vi "Cochlear Function Test Suite - Copy.vi"() -> ()   [LabVIEW 2020]
uses:
  CFTS SubVIs/CFTS-Globals.vi
  VsEP VIs/VsEP I-O Calibrator.vi
  ABR VIs/ABR Main Panel.vi
  ABR VIs/ABR3 Main Panel.vi
  CAPTH VIs/CAPTH Main Panel.vi
  DPOAE VIs/DP I-O (F1L1).vi
  DPOAE VIs/DP I-O Main Panel.vi
  Digital Exposure VIs/Digital Exposure Controller.vi
  RW Noise VIs/RW Noise VIs/RW Noise Controller.vi
  VsEP VIs/VsEP I-O Controller.vi
  DPOAE VIs/DP Analysis Panel.vi
  epl-vi-lib/Connection VIs/Connection Manager.vi
  System Test VIs/System Test.vi
  epl-cal-vi-lib/Calibrate Probe Tube.vi
  CAP Forward Masking/CAP Forward Masking.vi
  SFOAE VIs/SFOAE Main Panel.vi
  RW Noise VIs/PSTR VIs/PSTR Controller.vi
  epl-vi-lib/Utility VIs/File IO VIs/Configuration File Wrapper VIs/Config-Read Key (Boolean).vi
  epl-cal-vi-lib/Calibrate In Ear.vi
  <vilib>/Utility/miscctls.llb/LVStringsAndValuesArrayTypeDef_U16.ctl
  epl-vi-lib/Utility VIs/File IO VIs/Configuration File Wrapper VIs/Config-Read Key (string).vi
  CFTS SubVIs/CFTS-Experiment State.ctl
panel:
  in  "Other OAE":u16(ring) items=["Other OAE", "SFOAE", "SOAE"]
  in  "Undo":bool
  in  "Apply":bool
  in  "RW":u16(ring) items=["RW", "RW Noise", "PSTR"]
  in  "Other ABR":u16(ring) items=["Other ABR", "Masked ABR", "Fast ABR"]
  in  "Vitals":bool
  in  "Left":u16(ring) items=["---", "ABI-L", "ABI-R", "Insert Left", "Insert Right", "Left", "Right", "SN24", "SN31", "SN32", "SN36", "SN40", "SN41", "SN42"]
  in  "Right":u16(ring) items=["---", "ABI-L", "ABI-R", "Insert Left", "Insert Right", "Left", "Right", "SN24", "SN31", "SN32", "SN36", "SN40", "SN41", "SN42"]
  in  "CAP FM":bool caption="Boolean"
  in  "Options":bool
  in  "Expt State":T1 caption="Setup Options"
  in  "Help":bool
  in  "DP analysis":bool caption="Boolean"
  in  "Exposure":bool caption="Boolean"
  in  "System Test":bool
  in  "VsEP":bool caption="Boolean"
  out "VsEP Run#":i16
  in  "Connections":bool
  in  "VsEP Cal":bool
  in  "CAPTH":bool caption="Boolean"
  out "DP Run#":i16
  out "ABR Run#":i16
  out "CAP Run #":i16
  out "Data Folder":path
  in  "ABR":bool caption="Boolean"
  in  "DP I/O":bool caption="Boolean"
  in  "Calibrate in ear":bool
  in  "Calibrate probe tube":bool
  in  "Quit":bool caption="Boolean"
  # "EPL Cochlear Function Test Suite"
  # "Calibration"
  # "Measurements"
  # "Acoustic Systems"
  # "CTRL-A toggles advanced menu"
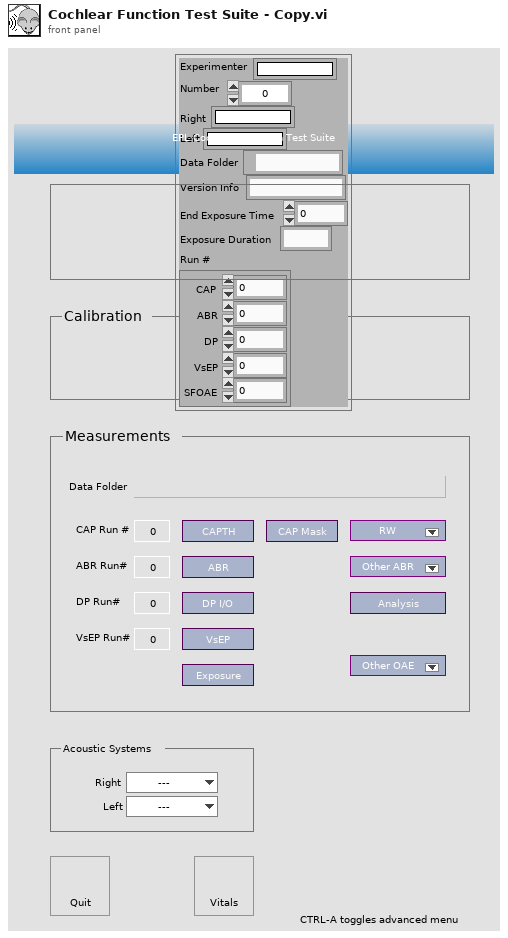
[diagram p1: front panel]
types:
  T1 = typedef "CFTS-Experiment State.ctl" = cluster{"Experimenter":string, "Number":u32, "Right":string, "Left":string, "Data Folder":path, "Version Info":string, "End Exposure Time":dbl, "Exposure Duration":string, "Run #":cluster{"CAP":i32, "ABR":i32, "DP":i32, "VsEP":i32, "SFOAE":i32}}
  T2 = typedef "LVStringsAndValuesArrayTypeDef_U16.ctl" = cluster{"String":string, "Value":u16}[]
  T3 = cluster{"CAP RUN #":refnum<vi>, "ABR RUN #":refnum<vi>, "DP RUN #":refnum<vi>, "VsEP RUN #":refnum<vi>}
  T4 = typedef "CFTS-Experiment State.ctl" = cluster{"Experimenter":string, "Number":u32, "Right":string, "Left":string, "Data Folder":path, "State File":path, "Version Info":string, "End Exposure Time":dbl, "Exposure Duration":string, "Run #":cluster{"CAP":i16, "ABR":i16, "DP":i16, "VsEP":i16, "MeasSeq":i16, "SubSeq":i16, "SFOAE":i16}}
  T5 = typedef "CFTS-Options.ctl" = cluster{"DP Artifact Rejection":bool, "Monitor vital signs ":bool, "Extension":string}
  T6 = cluster{"Experimenter":string, "Number":u32, "Right":string, "Left":string, "Data Folder":path, "State File":path, "Version Info":string, "End Exposure Time":dbl, "Exposure Duration":string, "Run #":cluster{"CAP":i16, "ABR":i16, "DP":i16, "VsEP":i16, "MeasSeq":i16, "SubSeq":i16, "SFOAE":i16}}
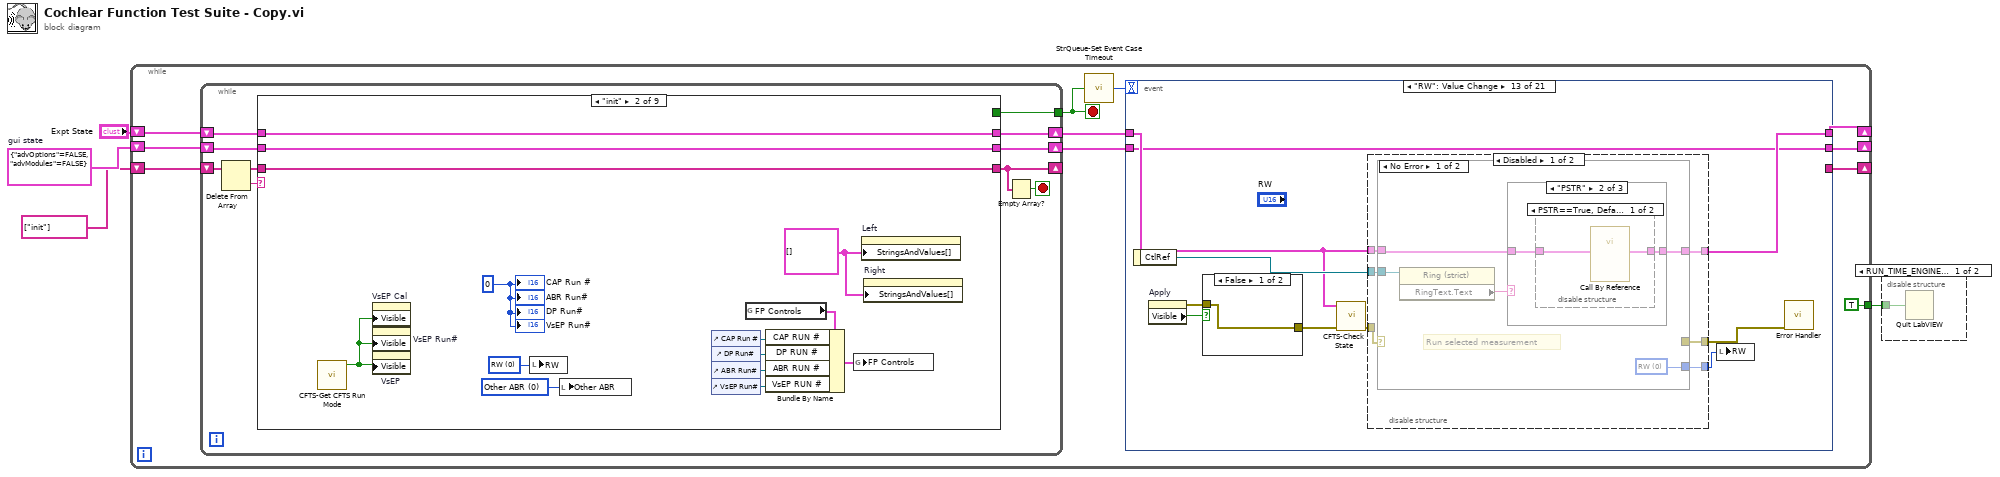
[diagram p0: block diagram]
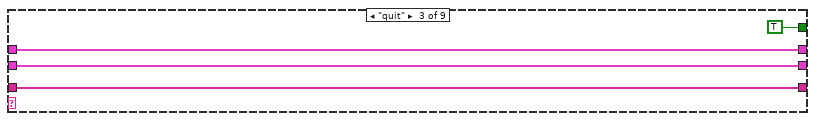
[diagram p3: hidden frame]
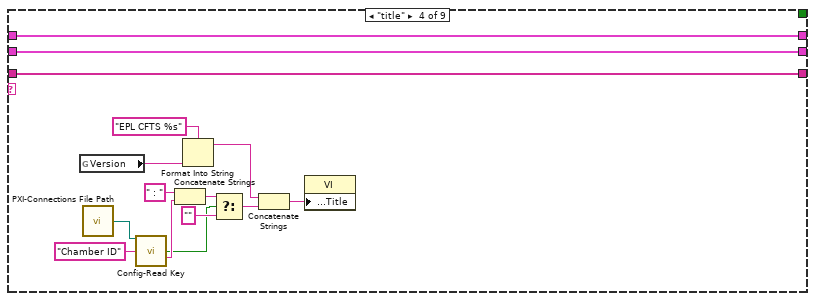
[diagram p4: hidden frame]
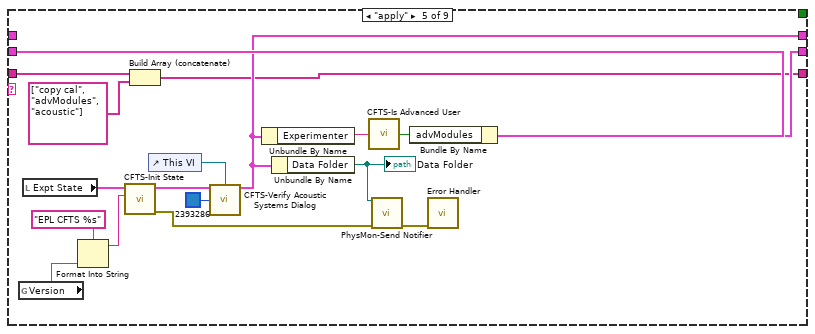
[diagram p5: hidden frame]
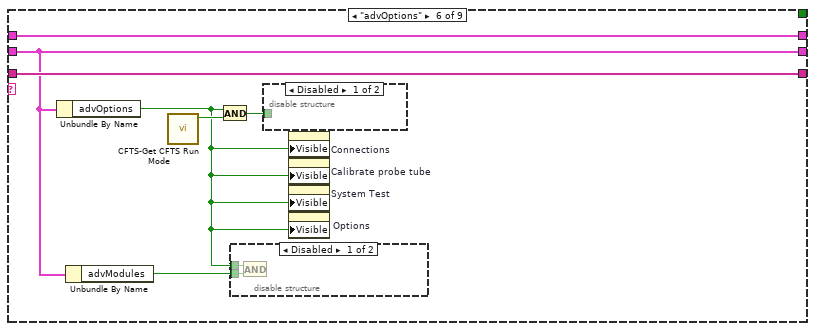
[diagram p6: hidden frame]
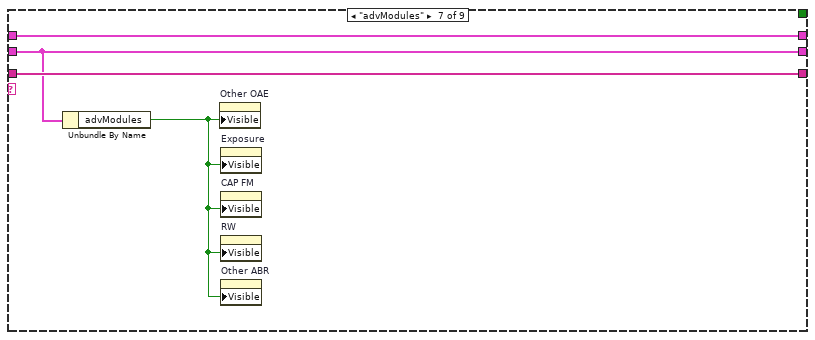
[diagram p9: hidden frame]
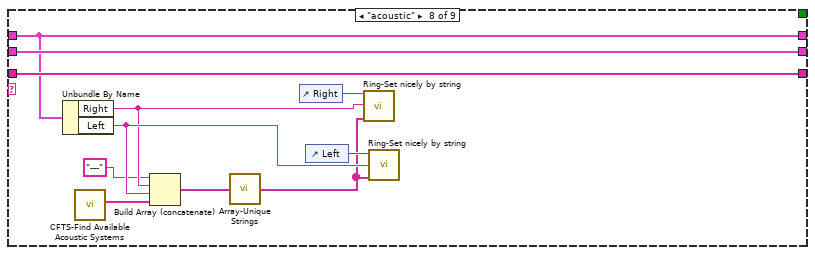
[diagram p10: hidden frame]
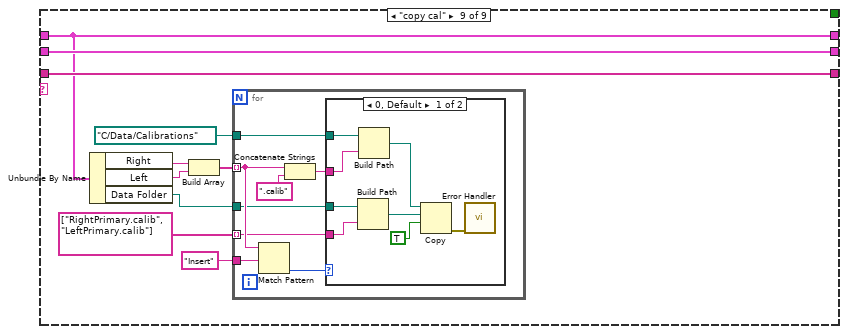
[diagram p11: hidden frame]
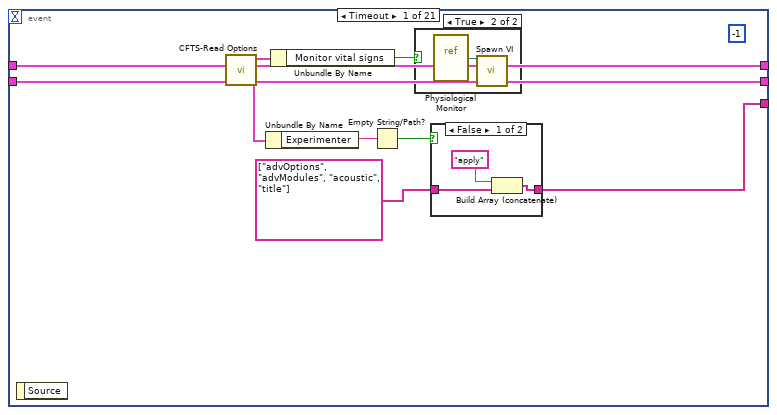
[diagram p13: hidden frame]
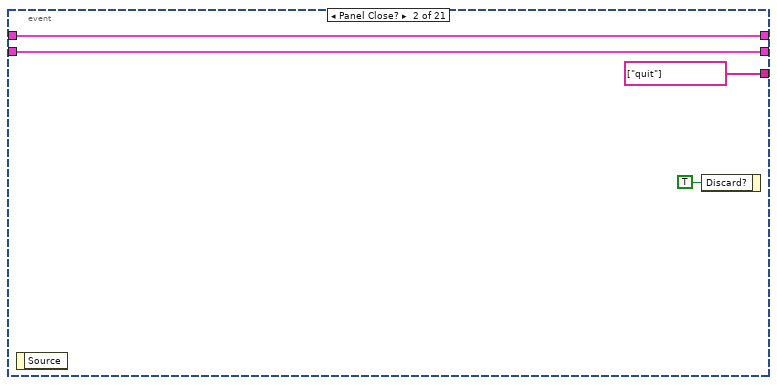
[diagram p16: hidden frame]
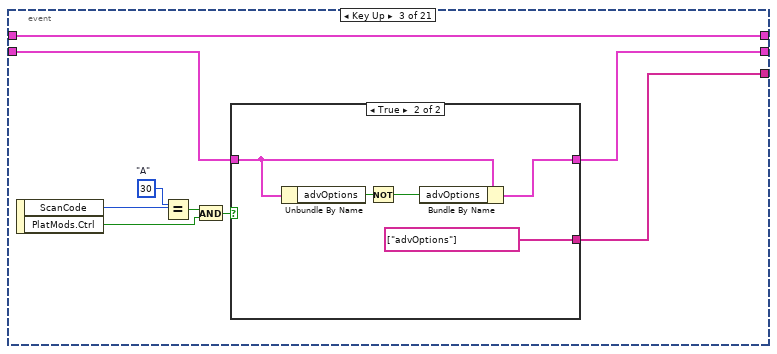
[diagram p17: hidden frame]
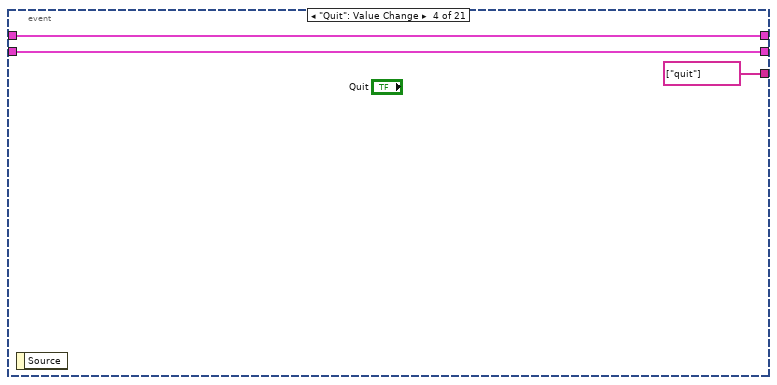
[diagram p19: hidden frame]
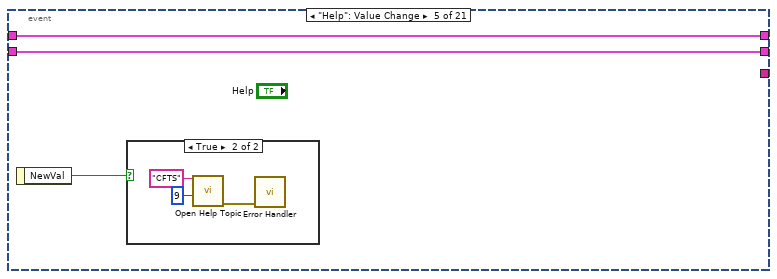
[diagram p20: hidden frame]
diagram:
  w2 = cluster{"advOptions":bool, "advModules":bool} {"advOptions"=FALSE, "advModules"=FALSE}  # gui state
  n1 = while {
    shift-right: [w10] -> _
    shift-left: "Expt State" -> [w14]
    tunnel: [TRUE] -> w3
    shift-right: [w9] -> _
    shift-left: w2 -> [w13]
    shift-right: [w5] -> _
    shift-left: string[] ["init"] ("Array") -> [w8]
    stop <- w6 stop-if-true
    n2 = while {
      shift-right: [w22] -> _
      shift-left: w8 -> [w25]
      tunnel: [w20] -> w6
      shift-right: [w19] -> w12
      shift-left: w14 -> [w18]
      shift-right: [w16] -> w11
      shift-left: w13 -> [w17]
      stop <- w21 stop-if-true
      n3 = Delete From Array(array=w25) -> (deleted portion=w23:string, array with subset deleted=w24:string[])  [unwired: 2 in]
      n4 = case shown="\"init\"" w23 {
        tunnel: w24 -> [w28 w42 w46 w61 w79 w86 w94 w105 w115]
        tunnel: [w28 w42 w46 w61 w67 w86 w94 w105 w115] -> w22
        tunnel: [_ _ TRUE _ _ _ _ _ _] -> w20
        tunnel: [w27 w41 w44 w60 w70 w85 w93 w103 w113] -> w19
        tunnel: w18 -> [w27 w41 w44 w60 _ w85 w93 w103 w113]
        tunnel: w17 -> [w26 w40 w43 w59 w78 w82 w92 w104 w114]
        tunnel: [w26 w40 w43 w59 w69 w82 w92 w104 w114] -> w16
        frame "", Default {
        }
        frame "init" {
          w29 = T2 [] ("Strings And Values []")
          w36 = i16 0 ("CAP RUN #")
          w38 = u16 0 items=["RW", "RW Noise", "PSTR"] ("RW")
          w37 = u16 0 items=["Other ABR", "Mask ABR", "Fast ABR"] ("Other ABR")
          n5 = call "CFTS-Get CFTS Run Mode.vi"() -> ("EPL Internal?"=w39:bool)  [unwired: 10 in, 1 out]
          n6 = property on="VsEP Cal" class="Bool"("Visible"=w39) -> ()  [unwired: 2 in, 2 out]
          n7 = property on="VsEP Run#" class="DigNum (strict)"("Visible"=w39) -> ()  [unwired: 2 in, 2 out]
          n8 = property on="VsEP" class="Bool"("Visible"=w39) -> ()  [unwired: 2 in, 2 out]
          n9 = local write "RW"(w38) -> ()
          n10 = local write "Other ABR"(w37) -> ()
          n11 = control-ref of="CAP Run #"() -> (w35:refnum<vi>)
          n12 = control-ref of="DP Run#"() -> (w34:refnum<vi>)
          n13 = control-ref of="ABR Run#"() -> (w33:refnum<vi>)
          n14 = control-ref of="VsEP Run#"() -> (w32:refnum<vi>)
          n15 = global read "CFTS-Globals.vi" "FP Controls"() -> (w30:T3)
          n16 = Bundle By Name(cluster=w30, "CAP RUN #"=w35, "DP RUN #"=w34, "ABR RUN #"=w33, "VsEP RUN #"=w32) -> (w31:T3)
          n17 = global write "CFTS-Globals.vi" "FP Controls"(w31) -> ()
          n18 = property on="Left" class="Ring (strict)"("StringsAndValues[]"=w29) -> ()  [unwired: 2 in, 2 out]
          n19 = property on="Right" class="Ring (strict)"("StringsAndValues[]"=w29) -> ()  [unwired: 2 in, 2 out]
          "CAP Run #" <- w36
          "ABR Run#" <- w36
          "DP Run#" <- w36
          "VsEP Run#" <- w36
        }
        frame "quit" {
        }
        frame "title" {
          n20 = global read "CFTS-Globals.vi" "Version"() -> (w47:string)
          n21 = call "PXI-Connections File Path.vi"() -> ("Path"=w58:path)  [unwired: 1 in]
          n22 = call-poly "Config-Read Key.vi"("configuration file path"=w58, "key"="Chamber ID" ("string")) -> ("found?"=w50:bool, "value"=w57:string)  [unwired: 10 in, 2 out]
          n23 = Concatenate Strings(" : " ("string"), w57) -> (w49:string)
          n24 = Format Into String(format string="EPL CFTS %s" ("string"), w47) -> (resulting string=w51:string)  [unwired: 2 in, 1 out]
          n25 = Select(t=w49, s=w50, f="") -> (s? t:f=w55:string)
          n26 = Concatenate Strings(w51, w55) -> (w52:string)
          n27 = property class="VI"("Front Panel.Title"=w52) -> ()  [unwired: 2 in, 2 out]
        }
        frame "apply" {
          n28 = global read "CFTS-Globals.vi" "Version"() -> (w62:string)
          n29 = local read "Expt State"() -> (w73:T1)
          n30 = Format Into String(format string="EPL CFTS %s" ("string"), w62) -> (resulting string=w63:string)  [unwired: 2 in, 1 out]
          n31 = call "CFTS-Init State.vi"("CFTS Version"=w63, "Experiment State (in)"=w73) -> ("error out"=w71:errorcluster, "Experiment State (out)"=w75:T4)  [unwired: 8 in]
          n32 = Build Array (concatenate)(w79, string[] ["copy cal", "advModules", "acoustic"]) -> (w67:string[])
          n33 = control-ref of="This VI"() -> (w76:refnum<vi>)
          n34 = call "CFTS-Verify Acoustic Systems Dialog.vi"("Expt State"=w75, "center on"=w76, "color"=u32 2393286) -> ("Cluster out"=w70:T1)  [unwired: 11 in, 1 out]
          n35 = Unbundle By Name(w70) -> ("Experimenter"=w74:string)
          n36 = Unbundle By Name(w70) -> ("Data Folder"=w65:path)
          "Data Folder" <- w65
          n37 = call "CFTS-Is Advanced User.vi"("Experimenter"=w74) -> ("Advanced user"=w68:bool)
          n38 = call "PhysMon-Send Notifier.vi"("Path"=w65, "error in (no error)"=w71) -> ("error out"=w72:errorcluster)  [unwired: 13 in]
          n39 = Bundle By Name(cluster=w78, "advModules"=w68) -> (w69:cluster{"advOptions":bool, "advModules":bool})
          n40 = call "Error Handler.vi"("error in (no error)"=w72) -> ()  [unwired: 13 in, 2 out]
        }
        frame "advOptions" {
          n41 = Unbundle By Name(w82) -> ("advOptions"=w81:bool)
          n42 = Unbundle By Name(w82) -> ("advModules"=w80:bool)
          n43 = call "CFTS-Get CFTS Run Mode.vi"() -> ("EPL Internal?"=w83:bool)  [unwired: 10 in, 1 out]
          n44 = And(x=w81, y=w83) -> (x .and. y?=w84:bool)
          n45 = disable-structure shown="Disabled" {
            disable-tunnel: w81 -> [w89 _]
            disable-tunnel: w80 -> [w88 _]
            frame Disabled {
              n46 = And(x=w89, y=w88) -> (x .and. y?=w90:bool)
            }
            frame Enabled {
            }
          }
          n47 = disable-structure shown="Disabled" {
            disable-tunnel: w84 -> [w87 _]
            frame Disabled {
            }
            frame Enabled {
            }
          }
          n48 = property on="Connections" class="Bool"("Visible"=w81) -> ()  [unwired: 2 in, 2 out]
          n49 = property on="Calibrate probe tube" class="Bool"("Visible"=w81) -> ()  [unwired: 2 in, 2 out]
          n50 = property on="System Test" class="Bool"("Visible"=w81) -> ()  [unwired: 2 in, 2 out]
          n51 = property on="Options" class="Bool"("Visible"=w81) -> ()  [unwired: 2 in, 2 out]
        }
        frame "advModules" {
          n52 = Unbundle By Name(w92) -> ("advModules"=w91:bool)
          n53 = property on="Other OAE" class="Ring (strict)"("Visible"=w91) -> ()  [unwired: 2 in, 2 out]
          n54 = property on="Exposure" class="Bool"("Visible"=w91) -> ()  [unwired: 2 in, 2 out]
          n55 = property on="CAP FM" class="Bool"("Visible"=w91) -> ()  [unwired: 2 in, 2 out]
          n56 = property on="RW" class="Ring (strict)"("Visible"=w91) -> ()  [unwired: 2 in, 2 out]
          n57 = property on="Other ABR" class="Ring (strict)"("Visible"=w91) -> ()  [unwired: 2 in, 2 out]
        }
        frame "acoustic" {
          n58 = Unbundle By Name(w103) -> ("Right"=w98:string, "Left"=w99:string)
          n59 = call "CFTS-Find Available Acoustic Systems.vi"() -> ("Acoustic Systems"=w100:string[])  [unwired: 11 in]
          n60 = Build Array (concatenate)("---", w98, w99, w100) -> (w96:string[])
          n61 = call "Array-Unique Strings.vi"("Strings"=w96) -> ("Unique strings"=w95:string[])  [unwired: 4 in]
          n62 = control-ref of="Right"() -> (w102:refnum<vi>)
          n63 = control-ref of="Left"() -> (w101:refnum<vi>)
          n64 = call "Ring-Set nicely by string.vi"("Ring in"=w102, "Device"=w98, "Strings []"=w95) -> ()  [unwired: 8 in, 5 out]
          n65 = call "Ring-Set nicely by string.vi"("Ring in"=w101, "Device"=w99, "Strings []"=w95) -> ()  [unwired: 8 in, 5 out]
        }
        frame "copy cal" {
          n66 = Unbundle By Name(w113) -> ("Right"=w112:string, "Left"=w111:string, "Data Folder"=w107:path)
          n67 = Build Array(w112, w111) -> (w110:string[])
          n68 = for {
            tunnel: w110 -> [w121] mode=indexing
            tunnel: "Insert" ("regular expression") -> [w123]
            tunnel: path "C:/Data/Calibrations" ("path") -> [w118]
            tunnel: w107 -> [w117]
            tunnel: string[] ["RightPrimary.calib", "LeftPrimary.calib"] ("regular expression") -> [w116] mode=indexing
            n69 = Match Pattern(string=w121, regular expression=w123) -> (offset past match=w122:i32)  [unwired: 1 in, 3 out]
            n70 = Concatenate Strings(w121, ".calib") -> (w119:string)
            n71 = case shown="0, Default" w122 {
              tunnel: w119 -> [w128 _]
              tunnel: w118 -> [w129 _]
              tunnel: w117 -> [w126 _]
              tunnel: w116 -> [w125 _]
              frame 0, Default {
                n72 = Build Path(base path=w126, name or relative path=w125) -> (appended path=w131:path)
                n73 = Build Path(base path=w129, name or relative path=w128) -> (appended path=w127:path)
                n74 = Copy(9:TRUE ("overwrite (F)"), 10:w131, 11:w127) -> (0:w130:errorcluster)  [unwired: 2 in, 2 out]
                n75 = call "Error Handler.vi"("error in (no error)"=w130) -> ()  [unwired: 13 in, 2 out]
              }
              frame -1 {
              }
            }
          }
        }
      }
      n76 = Empty Array?(array=w22) -> (empty?=w21:bool)
    }
    n77 = call "StrQueue-Set Event Case Timeout.vi"("Quit"=w6) -> ("timeout"=w7:i32)  [unwired: 14 in]
    n78 = event shown="[12] \"RW\": Value Change" {
      selector: _ -> [_ _ _ _ _ _ _ _ _ _ _ _ _ _ _ _ _ _ _ _ _]
      dyn-events: _ -> [_ _ _ _ _ _ _ _ _ _ _ _ _ _ _ _ _ _ _ _ _]
      timeout: w7 -> [_ _ _ _ _ _ _ _ _ _ _ _ _ _ _ _ _ _ _ _ _]
      tunnel: w12 -> [w136 w147 w152 w166 w169 w175 w178 w184 w189 w191 w201 w210 w260 w294 w325 w355 w359 w365 w372 w377 w383]
      tunnel: [w136 w147 w152 w166 w169 w175 w178 w184 w188 w191 w201 w216 w266 w300 w331 w355 w359 w362 w372 w377 w383] -> w10
      tunnel: [w132 string[] ["quit"] w149 string[] ["quit"] _ _ string[] ["apply"] _ _ _ _ _ _ _ _ _ _ string[] ["acoustic", "title"] _ string[] ["acoustic"] _] -> w5
      tunnel: [w137 w145 w150 w164 w167 w173 w177 w181 w185 w190 w200 w209 w258 w292 w323 w354 w358 w361 w371 w376 w382] -> w9
      tunnel: w11 -> [w137 w145 w151 w164 w167 w173 w177 w181 w185 w190 w200 w209 w258 w292 w323 w354 w358 w361 w371 w376 w382]
      event Timeout {
        (unwired) -1
        n79 = event-data() -> ()  [unwired: 1 in, 1 out]
        n80 = call "CFTS-Read Options.vi"() -> ("CFTS Options"=w139:T5)  [unwired: 10 in, 1 out]
        n81 = Unbundle By Name(w136) -> ("Experimenter"=w135:string)
        n82 = Unbundle By Name(w139) -> ("Monitor vital signs"=w138:bool)
        n83 = Empty String/Path?(string/path=w135) -> (empty?=w134:bool)
        n84 = case shown="True" w138 {
          frame False {
          }
          frame True {
            n85 = vi-ref "Physiological Monitor.vi"() -> (w144:refnum<vi>)
            n86 = call "Spawn VI.vi"("VI reference"=w144) -> ()  [unwired: 9 in, 2 out]
          }
        }
        n87 = case shown="False" w134 {
          tunnel: string[] ["advOptions", "advModules", "acoustic", "title"] -> [w142 w143]
          tunnel: [w141 w143] -> w132
          frame False {
            n88 = Build Array (concatenate)("apply", w142) -> (w141:string[])
          }
          frame True {
          }
        }
      }
      event Panel Close? {
        n89 = event-data() -> ()  [unwired: 1 in, 1 out]
        n90 = event-data("Discard?"=TRUE) -> ()  [unwired: 1 in, 1 out]
      }
      event Key Up {
        w156 = i16 30  # "A"
        n91 = event-data() -> ("ScanCode"=w157:i16, "PlatMods.Ctrl"=w154:bool)  [unwired: 1 in]
        n92 = Equal?(x=w156, y=w157) -> (x = y?=w155:bool)
        n93 = And(x=w155, y=w154) -> (x .and. y?=w153:bool)
        n94 = case shown="True" w153 {
          tunnel: w151 -> [w158 w163]
          tunnel: [w158 w160] -> w150
          tunnel: [_ string[] ["advOptions"]] -> w149
          frame False {
          }
          frame True {
            n95 = Unbundle By Name(w163) -> ("advOptions"=w162:bool)
            n96 = Not(x=w162) -> (.not. x?=w161:bool)
            n97 = Bundle By Name(cluster=w163, "advOptions"=w161) -> (w160:cluster{"advOptions":bool, "advModules":bool})
          }
        }
      }
      event "Quit": Value Change {
        n98 = event-data() -> ()  [unwired: 1 in, 1 out]
      }
      event "Help": Value Change {
        n99 = event-data() -> ("NewVal"=w168:bool)  [unwired: 1 in]
        n100 = case shown="True" w168 {
          frame False {
          }
          frame True {
            n101 = call "Open Help Topic.vi"("Help file"="CFTS", "HelpId"=9) -> ("error out"=w171:errorcluster)  [unwired: 13 in]
            n102 = call "Error Handler.vi"("error in (no error)"=w171) -> ()  [unwired: 13 in, 2 out]
          }
        }
      }
      event Value Change {
        w174 = TRUE ("Visible")
        n103 = event-data() -> ()  [unwired: 1 in, 1 out]
        n104 = property on="Undo" class="Bool"("Visible"=w174) -> ()  [unwired: 2 in, 2 out]
        n105 = property on="Apply" class="Bool"("Visible"=w174) -> ()  [unwired: 2 in, 2 out]
      }
      event "Apply": Value Change {
        w179 = FALSE
        n106 = event-data() -> ()  [unwired: 1 in, 1 out]
        n107 = property on="Apply" class="Bool"("Visible"=w179) -> (error out=w180:errorcluster)  [unwired: 2 in, 1 out]
        n108 = property on="Undo" class="Bool"(error in=w180, "Visible"=w179) -> ()  [unwired: 1 in, 2 out]
      }
      event "Undo": Value Change {
        w183 = FALSE
        n109 = event-data() -> ()  [unwired: 1 in, 1 out]
        n110 = local write "Expt State"(w184) -> ()
        n111 = property on="Apply" class="Bool"("Visible"=w183) -> (error out=w182:errorcluster)  [unwired: 2 in, 1 out]
        n112 = property on="Undo" class="Bool"(error in=w182, "Visible"=w183) -> ()  [unwired: 1 in, 2 out]
      }
      event "Right", "Left": Value Change {
        n113 = event-data() -> ()  [unwired: 1 in, 1 out]
        n114 = property on="Left" class="Ring (strict)"() -> ("RingText.Text"=w187:string)  [unwired: 2 in, 2 out]
        n115 = property on="Right" class="Ring (strict)"() -> ("RingText.Text"=w186:string)  [unwired: 2 in, 2 out]
        n116 = Bundle By Name(cluster=w189, "Right"=w186, "Left"=w187) -> (w188:T1)
        n117 = call "CFTS-Store Acoustic System IDs.vi"("Left"=w187, "Right"=w186) -> ()  [unwired: 9 in, 1 out]
      }
      event "Calibrate in ear": Value Change {
        n118 = event-data() -> ()  [unwired: 1 in, 1 out]
        n119 = disable-structure shown="Disabled" {
          disable-tunnel: w191 -> [w193 _]
          frame Disabled {
            n120 = call "CFTS-Check State.vi"("Expt State"=w193) -> ("error out"=w194:errorcluster)  [unwired: 10 in]
            n121 = case shown="No Error" w194 {
              selector: w194 -> [_ w199]
              tunnel: w193 -> [w198 _]
              tunnel: [w197 w199] -> w192
              frame No Error {
                n122 = call "PXI-Connections File Path.vi"() -> ("Path"=w196:path)  [unwired: 1 in]
                n123 = call-poly "Config-Read Key.vi"("configuration file path"=w196, "key"="FPL") -> ()  [unwired: 10 in, 4 out]
                n124 = call-by-ref "?"("State"=w198) -> ("error out"=w197:errorcluster)  [unwired: 12 in, 2 out]
              }
              frame Error {
              }
            }
            n125 = call "Error Handler.vi"("error in (no error)"=w192) -> ()  [unwired: 13 in, 2 out]
          }
          frame Enabled {
          }
        }
      }
      event "VsEP Cal": Value Change {
        n126 = event-data() -> ()  [unwired: 1 in, 1 out]
        n127 = disable-structure shown="Disabled" {
          disable-tunnel: w201 -> [w204 _]
          frame Disabled {
            n128 = call "CFTS-Check State.vi"("Expt State"=w204) -> ("error out"=w203:errorcluster)  [unwired: 10 in]
            n129 = Unbundle By Name(w204) -> ("Data Folder"=w205:path)
            n130 = case shown="No Error" w203 {
              selector: w203 -> [w206 w208]
              tunnel: w205 -> [w207 _]
              tunnel: [w206 w208] -> w202
              frame No Error {
                n131 = call-by-ref "?"("Data Folder"=w207) -> ()  [unwired: 13 in, 2 out]
              }
              frame Error {
              }
            }
            n132 = call "Error Handler.vi"("error in (no error)"=w202) -> ()  [unwired: 13 in, 2 out]
          }
          frame Enabled {
          }
        }
      }
      event "DP I/O", "ABR", "CAPTH", "VsEP", "Exposure", "CAP FM": Value Change {
        n133 = event-data() -> ("CtlRef"=w217:refnum<vi>)  [unwired: 1 in]
        n134 = property on="Apply" class="Bool"() -> (error out=w213:errorcluster, "Visible"=w214:bool)  [unwired: 2 in, 1 out]
        n135 = case shown="True" w214 {
          tunnel: w213 -> [w255 _]
          tunnel: [w255 w256] -> w212
          frame False {
          }
          frame True {
            n136 = call <vilib>:"Error Cluster From Error Code.vi"("error code (0)"=5001) -> ("error out"=w256:errorcluster)  [unwired: 8 in]
          }
        }
        n137 = call "CFTS-Check State.vi"("error in (no error)"=w212, "Expt State"=w210) -> ("error out"=w211:errorcluster)  [unwired: 9 in]
        n138 = disable-structure shown="Disabled" {
          disable-tunnel: w217 -> [w222 _]
          disable-tunnel: [w221 _] -> w216
          disable-tunnel: [w220 _] -> w215
          disable-tunnel: w211 -> [w219 _]
          disable-tunnel: w210 -> [w218 _]
          frame Disabled {
            n139 = case shown="No Error" w219 {
              selector: w219 -> [_ w253]
              tunnel: w222 -> [w226 _]
              tunnel: w218 -> [w224 w254]
              tunnel: [w223 w254] -> w221
              tunnel: [_ w253] -> w220
              frame No Error {
                # "Run selected measurement"
                n140 = property class="Bool"(reference=w226) -> ("Label.Text"=w225:string)  [unwired: 1 in, 2 out]
                n141 = case shown="\"CAPTH\"" w225 {
                  tunnel: w224 -> [w228 w230 w232 w240 w246 w248 w250 w252]
                  tunnel: [w227 w229 w231 w239 w245 w247 w249 w251] -> w223
                  frame "ABR" {
                    n142 = call-by-ref "?"("State (in)"=w228) -> ("State"=w227:T4)  [unwired: 12 in, 2 out]
                  }
                  frame "CAP FM" {
                    n143 = call-by-ref "?"("State"=w230) -> ("State Out"=w229:T4)  [unwired: 12 in, 2 out]
                  }
                  frame "CAPTH" {
                    n144 = disable-structure shown="Enabled" {
                      disable-tunnel: w232 -> [w234 w235]
                      disable-tunnel: [w233 w235] -> w231
                      frame Enabled {
                        n145 = call-by-ref "?"("Expt State (in)"=w234) -> ("State"=w233:T4)  [unwired: 12 in, 2 out]
                      }
                      frame Disabled {
                      }
                    }
                  }
                  frame "DP I/O", Default {
                    n146 = call "PXI-Connections File Path.vi"() -> ("Path"=w236:path)  [unwired: 1 in]
                    n147 = call-poly "Config-Read Key.vi"("configuration file path"=w236, "key"="Advanced DP I-O") -> ("value"=w237:bool)  [unwired: 10 in, 3 out]
                    n148 = case shown="False" w237 {
                      tunnel: w240 -> [w242 w244]
                      tunnel: [w241 w243] -> w239
                      frame True {
                        n149 = call-by-ref "?"("Expt State (in)"=w242) -> ("State"=w241:T4)  [unwired: 12 in, 2 out]
                      }
                      frame False {
                        n150 = call-by-ref "?"("Expt State (in)"=w244) -> ("State"=w243:T4)  [unwired: 12 in, 2 out]
                      }
                    }
                  }
                  frame "Exposure" {
                    n151 = call-by-ref "?"("State in"=w246) -> ("State"=w245:T4)  [unwired: 12 in, 2 out]
                  }
                  frame "Masked ABR" {
                    n152 = call-by-ref "?"("State (in)"=w248) -> ("State"=w247:T4)  [unwired: 12 in, 2 out]
                  }
                  frame "RW Noise" {
                    n153 = call-by-ref "?"("Expt State (in)"=w250) -> ("Expt State"=w249:T4)  [unwired: 12 in, 2 out]
                  }
                  frame "VsEP" {
                    n154 = call-by-ref "?"("Expt State (in)"=w252) -> ("state out"=w251:T4)  [unwired: 12 in, 2 out]
                  }
                }
              }
              frame Error {
              }
            }
          }
          frame Enabled {
          }
        }
        n155 = call "Error Handler.vi"("error in (no error)"=w215) -> ()  [unwired: 13 in, 2 out]
      }
      event "RW": Value Change {
        n156 = event-data() -> ("CtlRef"=w267:refnum<vi>)  [unwired: 1 in]
        n157 = property on="Apply" class="Bool"() -> (error out=w263:errorcluster, "Visible"=w264:bool)  [unwired: 2 in, 1 out]
        n158 = case shown="False" w264 {
          tunnel: w263 -> [w289 _]
          tunnel: [w289 w290] -> w262
          frame False {
          }
          frame True {
            n159 = call <vilib>:"Error Cluster From Error Code.vi"("error code (0)"=5001) -> ("error out"=w290:errorcluster)  [unwired: 8 in]
          }
        }
        n160 = call "CFTS-Check State.vi"("error in (no error)"=w262, "Expt State"=w260) -> ("error out"=w261:errorcluster)  [unwired: 9 in]
        n161 = disable-structure shown="Disabled" {
          disable-tunnel: w267 -> [w273 _]
          disable-tunnel: [w272 _] -> w266
          disable-tunnel: [w271 _] -> w265
          disable-tunnel: w261 -> [w270 _]
          disable-tunnel: w260 -> [w269 _]
          disable-tunnel: [w268 _] -> w259
          frame Disabled {
            n162 = case shown="No Error" w270 {
              selector: w270 -> [_ w287]
              tunnel: w273 -> [w278 _]
              tunnel: w269 -> [w276 w288]
              tunnel: [w275 w288] -> w272
              tunnel: [_ w287] -> w271
              tunnel: [w274 _] -> w268
              frame No Error {
                w274 = u16 0 items=["RW", "RW Noise", "PSTR"] ("RW")
                # "Run selected measurement"
                n163 = property class="Ring (strict)"(reference=w278) -> ("RingText.Text"=w277:string)  [unwired: 1 in, 2 out]
                n164 = case shown="\"PSTR\"" w277 {
                  tunnel: w276 -> [w279 w280 w286]
                  tunnel: [w279 w281 w285] -> w275
                  frame "", Default {
                  }
                  frame "PSTR" {
                    n165 = disable-structure shown="PSTR==True, Default" {
                      disable-tunnel: [w283 w284] -> w281
                      disable-tunnel: w280 -> [w282 w284]
                      frame condition #0 (active) {
                        n166 = call-by-ref "?"("Expt State (in)"=w282) -> ("Expt State"=w283:T4)  [unwired: 12 in, 2 out]
                      }
                      frame condition #1 {
                      }
                    }
                  }
                  frame "RW Noise" {
                    n167 = call-by-ref "?"("Expt State (in)"=w286) -> ("Expt State"=w285:T4)  [unwired: 12 in, 2 out]
                  }
                }
              }
              frame Error {
              }
            }
          }
          frame Enabled {
          }
        }
        n168 = local write "RW"(w259) -> ()
        n169 = call "Error Handler.vi"("error in (no error)"=w265) -> ()  [unwired: 13 in, 2 out]
      }
      event "Other ABR": Value Change {
        n170 = event-data() -> ("CtlRef"=w301:refnum<vi>)  [unwired: 1 in]
        n171 = property on="Apply" class="Bool"() -> (error out=w297:errorcluster, "Visible"=w298:bool)  [unwired: 2 in, 1 out]
        n172 = case shown="True" w298 {
          tunnel: w297 -> [w320 _]
          tunnel: [w320 w321] -> w296
          frame False {
          }
          frame True {
            n173 = call <vilib>:"Error Cluster From Error Code.vi"("error code (0)"=5001) -> ("error out"=w321:errorcluster)  [unwired: 8 in]
          }
        }
        n174 = call "CFTS-Check State.vi"("error in (no error)"=w296, "Expt State"=w294) -> ("error out"=w295:errorcluster)  [unwired: 9 in]
        n175 = disable-structure shown="Disabled" {
          disable-tunnel: w301 -> [w307 _]
          disable-tunnel: [w306 _] -> w300
          disable-tunnel: [w305 _] -> w299
          disable-tunnel: w295 -> [w304 _]
          disable-tunnel: w294 -> [w303 _]
          disable-tunnel: [w302 _] -> w293
          frame Disabled {
            n176 = case shown="No Error" w304 {
              selector: w304 -> [_ w318]
              tunnel: w307 -> [w312 _]
              tunnel: w303 -> [w310 w319]
              tunnel: [w309 w319] -> w306
              tunnel: [_ w318] -> w305
              tunnel: [0 _] -> w302
              frame No Error {
                # "Run selected measurement"
                n177 = property class="Ring (strict)"(reference=w312) -> ("RingText.Text"=w311:string)  [unwired: 1 in, 2 out]
                n178 = case shown="\"Masked ABR\"" w311 {
                  tunnel: w310 -> [w314 w315 w316]
                  tunnel: [w313 w315 w317] -> w309
                  frame "Masked ABR" {
                    n179 = call-by-ref "?"("State (in)"=w314) -> ("State"=w313:T4)  [unwired: 12 in, 2 out]
                  }
                  frame "", Default {
                  }
                  frame "Fast ABR" {
                    n180 = call "Fast ABR.vi"("Expt State (in)"=w316) -> ("Expt State"=w317:T4)  [unwired: 10 in]
                  }
                }
              }
              frame Error {
              }
            }
          }
          frame Enabled {
          }
        }
        n181 = local write "Other ABR"(w293) -> ()
        n182 = call "Error Handler.vi"("error in (no error)"=w299) -> ()  [unwired: 13 in, 2 out]
      }
      event "Other OAE": Value Change {
        n183 = event-data() -> ("CtlRef"=w332:refnum<vi>)  [unwired: 1 in]
        n184 = property on="Apply" class="Bool"() -> (error out=w328:errorcluster, "Visible"=w329:bool)  [unwired: 2 in, 1 out]
        n185 = case shown="True" w329 {
          tunnel: w328 -> [w351 _]
          tunnel: [w351 w352] -> w327
          frame False {
          }
          frame True {
            n186 = call <vilib>:"Error Cluster From Error Code.vi"("error code (0)"=5001) -> ("error out"=w352:errorcluster)  [unwired: 8 in]
          }
        }
        n187 = call "CFTS-Check State.vi"("error in (no error)"=w327, "Expt State"=w325) -> ("error out"=w326:errorcluster)  [unwired: 9 in]
        n188 = disable-structure shown="Disabled" {
          disable-tunnel: w332 -> [w338 _]
          disable-tunnel: [w337 _] -> w331
          disable-tunnel: [w336 _] -> w330
          disable-tunnel: w326 -> [w335 _]
          disable-tunnel: w325 -> [w334 _]
          disable-tunnel: [w333 _] -> w324
          frame Disabled {
            n189 = case shown="No Error" w335 {
              selector: w335 -> [_ w349]
              tunnel: w338 -> [w343 _]
              tunnel: w334 -> [w341 w350]
              tunnel: [w340 w350] -> w337
              tunnel: [_ w349] -> w336
              tunnel: [0 _] -> w333
              frame No Error {
                # "Run selected measurement"
                n190 = property class="Ring (strict)"(reference=w343) -> ("RingText.Text"=w342:string)  [unwired: 1 in, 2 out]
                n191 = case shown="\"SOAE\"" w342 {
                  tunnel: w341 -> [w344 w346 w348]
                  tunnel: [w344 w345 w347] -> w340
                  frame "", Default {
                  }
                  frame "SFOAE" {
                    n192 = call-by-ref "?"("Expt State (in)"=w346) -> ("State"=w345:T6)  [unwired: 12 in, 2 out]
                  }
                  frame "SOAE" {
                    n193 = call "SOAE Main Panel.vi"("Expt State (in)"=w348) -> ("Expt State out"=w347:T4)  [unwired: 14 in]
                  }
                }
              }
              frame Error {
              }
            }
          }
          frame Enabled {
          }
        }
        n194 = local write "Other OAE"(w324) -> ()
        n195 = call "Error Handler.vi"("error in (no error)"=w330) -> ()  [unwired: 13 in, 2 out]
      }
      event "DP analysis": Value Change {
        n196 = event-data() -> ()  [unwired: 1 in, 1 out]
        n197 = disable-structure shown="Disabled" {
          disable-tunnel: w355 -> [w357 _]
          frame Disabled {
            n198 = Unbundle By Name(w357) -> ("Data Folder"=w356:path)
            n199 = call-by-ref "?"("Data folder in"=w356) -> ()  [unwired: 13 in, 2 out]
          }
          frame Enabled {
          }
        }
      }
      event "Connections": Value Change {
        n200 = event-data() -> ()  [unwired: 1 in, 1 out]
        n201 = disable-structure shown="Disabled" {
          frame Disabled {
            n202 = call-by-ref "?"() -> ()  [unwired: 14 in, 2 out]
          }
          frame Enabled {
          }
        }
      }
      event "Options": Value Change {
        n203 = event-data() -> ()  [unwired: 1 in, 1 out]
        n204 = disable-structure shown="Disabled" {
          disable-tunnel: [w370 _] -> w364
          disable-tunnel: [w369 _] -> w363
          frame Disabled {
            n205 = call "CFTS-Get Acoustic System IDs.vi"() -> ("error out"=w366:errorcluster, "Left"=w368:string, "Right"=w367:string)  [unwired: 9 in]
            n206 = call "CFTS-Options Dialog.vi"("Left"=w368, "Right"=w367) -> ("Left out"=w369:string, "Right out"=w370:string)  [unwired: 7 in, 1 out]
            n207 = call "CFTS-Store Acoustic System IDs.vi"("error in (no error)"=w366, "Left"=w369, "Right"=w370) -> ()  [unwired: 8 in, 1 out]
          }
          frame Enabled {
          }
        }
        n208 = Bundle By Name(cluster=w365, "Right"=w364, "Left"=w363) -> (w362:T1)
      }
      event "System Test": Value Change {
        n209 = event-data() -> ()  [unwired: 1 in, 1 out]
        n210 = disable-structure shown="Disabled" {
          disable-tunnel: w372 -> [w374 _]
          frame Disabled {
            n211 = Unbundle By Name(w374) -> ("Data Folder"=w373:path)
            n212 = call-by-ref "?"("Data Folder"=w373) -> ()  [unwired: 13 in, 2 out]
          }
          frame Enabled {
          }
        }
      }
      event "Calibrate probe tube": Value Change {
        n213 = event-data() -> ()  [unwired: 1 in, 1 out]
        n214 = disable-structure shown="Disabled" {
          disable-tunnel: w377 -> [w379 _]
          frame Disabled {
            n215 = Unbundle By Name(w379) -> ("Experimenter"=w378:string, "Right"=w381:string, "Left"=w380:string)
            n216 = call-by-ref "?"("Left"=w380, "Right"=w381, "User ID"=w378) -> ()  [unwired: 11 in, 2 out]
          }
          frame Enabled {
          }
        }
      }
      event "Vitals": Value Change {
        n217 = event-data() -> ()  [unwired: 1 in, 1 out]
        n218 = disable-structure shown="Disabled" {
          disable-tunnel: w383 -> [w387 _]
          frame Disabled {
            n219 = vi-ref "Physiological Monitor.vi"() -> (w389:refnum<vi>)
            n220 = Unbundle By Name(w387) -> ("Data Folder"=w386:path)
            n221 = call "Spawn VI.vi"("VI reference"=w389) -> ("error out"=w388:errorcluster, "Started?"=w385:bool)  [unwired: 9 in]
            n222 = case shown="True" w385 {
              tunnel: w388 -> [w390 w393]
              tunnel: w386 -> [_ w392]
              tunnel: [w390 w391] -> w384
              frame False {
              }
              frame True {
                n223 = call "PhysMon-Send Notifier.vi"("Path"=w392, "error in (no error)"=w393) -> ("error out"=w391:errorcluster)  [unwired: 13 in]
              }
            }
            n224 = call "Error Handler.vi"("error in (no error)"=w384) -> ()  [unwired: 13 in, 2 out]
          }
          frame Enabled {
          }
        }
      }
    }
  }
  n225 = disable-structure shown="RUN_TIME_ENGINE==True" {
    disable-tunnel: w3 -> [w394 _]
    frame condition #0 {
      n226 = Quit LabVIEW(quit? (T)=w394) -> ()
    }
    frame condition #1 (active) {
    }
  }
